vi "checkplayerstatus.vi"(11 "player":T1[](array[typedef]) {"status" items=["host_ready", "idle", "host", "leaved", "ready", "playing", "lose(mine)", "lose(ot)", "win"]}) -> (3 "Numeric":u16, 7 "kick leave":T1[](array[typedef]) {"status" items=["host_ready", "idle", "host", "leaved", "ready", "playing", "lose(mine)", "lose(ot)", "win"]})   [LabVIEW 2025]
uses:
  controls/playerstatus.ctl
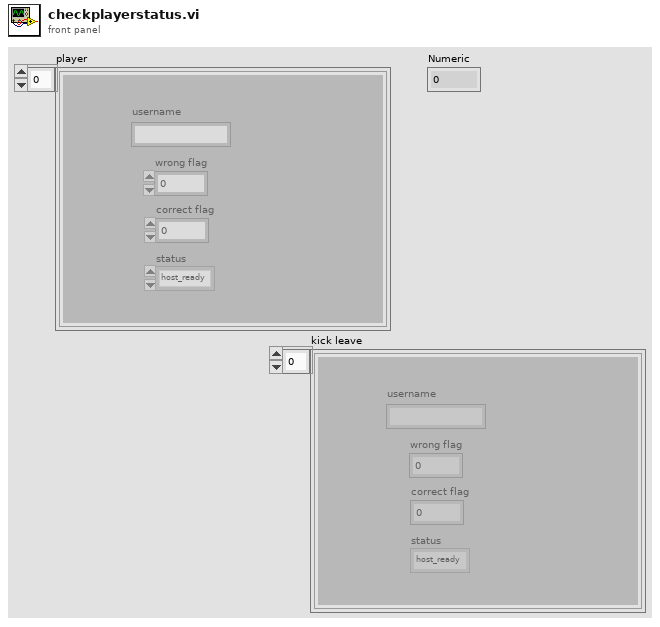
[diagram p1: front panel]
types:
  T1 = typedef "playerstatus.ctl" = cluster{"correct flag":i32, "wrong flag":i32, "username":string, "status":u16}
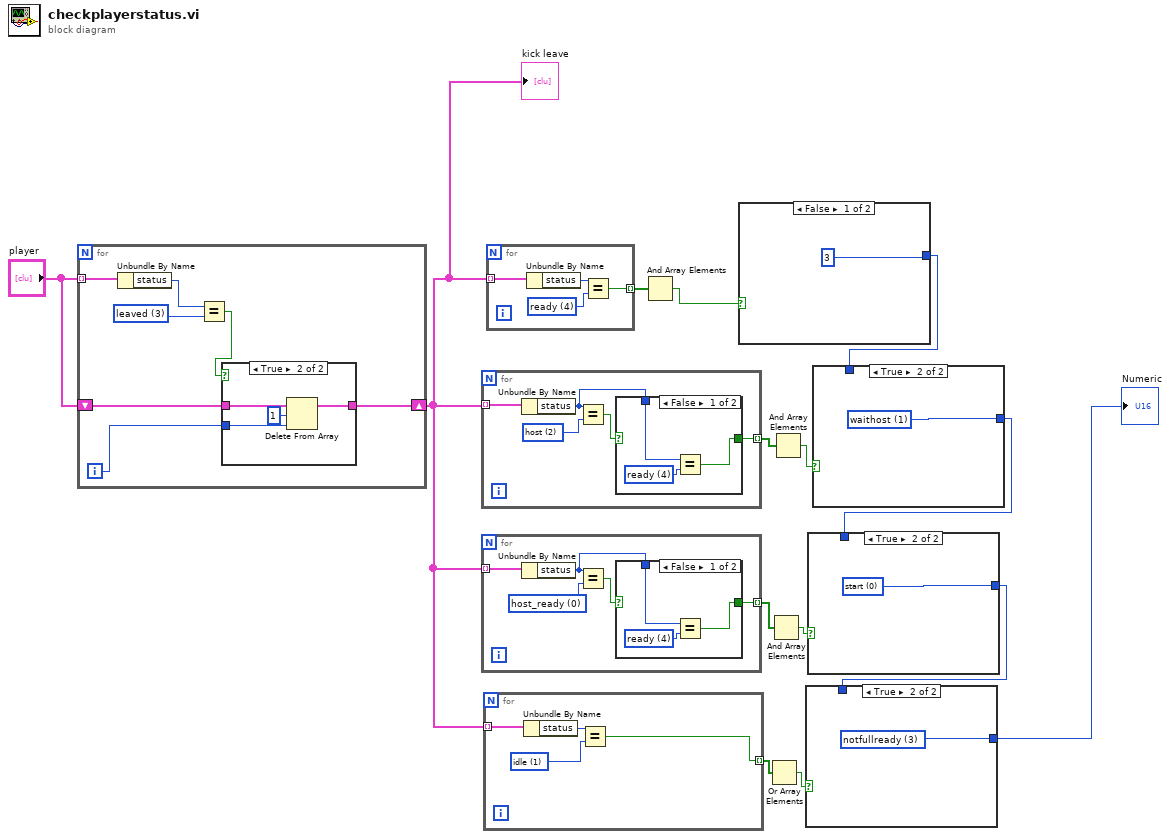
[diagram p0: block diagram]
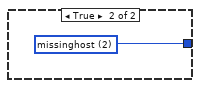
[diagram p7: hidden frame]
diagram:
  n1 = for {
    tunnel: "player" -> [w20] mode=indexing
    shift-right: [w15] -> w1
    shift-left: "player" -> [w18]
    i -> [w16]
    w19 = u16 3 items=["host_ready", "idle", "host", "leaved", "ready", "playing", "lose(mine)", "lose(ot)", "win"] ("status")
    n2 = Unbundle By Name(w20) -> ("status"=w21:u16)
    n3 = Equal?(x=w21, y=w19) -> (x = y?=w17:bool)
    n4 = case shown="True" w17 {
      tunnel: w18 -> [w22 w26]
      tunnel: w16 -> [_ w25]
      tunnel: [w22 w23] -> w15
      frame False {
      }
      frame True {
        n5 = Delete From Array(array=w26, length=1, index=w25) -> (array with subset deleted=w23:T1[])  [unwired: 1 out]
      }
    }
  }
  "kick leave" <- w1
  n6 = for {
    tunnel: w1 -> [w31] mode=indexing
    tunnel: [w28] -> w11 mode=indexing
    w30 = u16 2 items=["host_ready", "idle", "host", "leaved", "ready", "playing", "lose(mine)", "lose(ot)", "win"] ("status")
    n7 = Unbundle By Name(w31) -> ("status"=w27:u16)
    n8 = Equal?(x=w27, y=w30) -> (x = y?=w29:bool)
    n9 = case shown="False" w29 {
      selector: w29 -> [_ w35]
      tunnel: [w32 w35] -> w28
      tunnel: w27 -> [w34 _]
      frame False {
        w33 = u16 4 items=["host_ready", "idle", "host", "leaved", "ready", "playing", "lose(mine)", "lose(ot)", "win"] ("status")
        n10 = Equal?(x=w34, y=w33) -> (x = y?=w32:bool)
      }
      frame True {
      }
    }
  }
  n11 = for {
    tunnel: w1 -> [w40] mode=indexing
    tunnel: [w37] -> w7 mode=indexing
    w39 = u16 0 items=["host_ready", "idle", "host", "leaved", "ready", "playing", "lose(mine)", "lose(ot)", "win"] ("status")
    n12 = Unbundle By Name(w40) -> ("status"=w36:u16)
    n13 = Equal?(x=w36, y=w39) -> (x = y?=w38:bool)
    n14 = case shown="False" w38 {
      selector: w38 -> [_ w44]
      tunnel: [w41 w44] -> w37
      tunnel: w36 -> [w43 _]
      frame False {
        w42 = u16 4 items=["host_ready", "idle", "host", "leaved", "ready", "playing", "lose(mine)", "lose(ot)", "win"] ("status")
        n15 = Equal?(x=w43, y=w42) -> (x = y?=w41:bool)
      }
      frame True {
      }
    }
  }
  n16 = for {
    tunnel: w1 -> [w48] mode=indexing
    tunnel: [w45] -> w5 mode=indexing
    w47 = u16 1 items=["host_ready", "idle", "host", "leaved", "ready", "playing", "lose(mine)", "lose(ot)", "win"] ("status")
    n17 = Unbundle By Name(w48) -> ("status"=w46:u16)
    n18 = Equal?(x=w46, y=w47) -> (x = y?=w45:bool)
  }
  n19 = for {
    tunnel: w1 -> [w52] mode=indexing
    tunnel: [w49] -> w13 mode=indexing
    w50 = u16 4 items=["host_ready", "idle", "host", "leaved", "ready", "playing", "lose(mine)", "lose(ot)", "win"] ("status")
    n20 = Unbundle By Name(w52) -> ("status"=w51:u16)
    n21 = Equal?(x=w51, y=w50) -> (x = y?=w49:bool)
  }
  n22 = And Array Elements(Boolean array=w13) -> (logical AND=w12:bool)
  n23 = case shown="False" w12 {
    tunnel: [u16 3 w54] -> w9
    frame False {
    }
    frame True {
      w54 = u16 2 items=["start", "waithost", "missinghost", "notfullready"]
    }
  }
  n24 = Or Array Elements(Boolean array=w5) -> (logical OR=w4:bool)
  n25 = And Array Elements(Boolean array=w7) -> (logical AND=w6:bool)
  n26 = And Array Elements(Boolean array=w11) -> (logical AND=w10:bool)
  n27 = case shown="True" w10 {
    tunnel: [w55 w56] -> w8
    tunnel: w9 -> [w55 _]
    frame False {
    }
    frame True {
      w56 = u16 1 items=["start", "waithost", "missinghost", "notfullready"]
    }
  }
  n28 = case shown="True" w6 {
    tunnel: [w57 w58] -> w3
    tunnel: w8 -> [w57 _]
    frame False {
    }
    frame True {
      w58 = u16 0 items=["start", "waithost", "missinghost", "notfullready"]
    }
  }
  n29 = case shown="True" w4 {
    tunnel: [w59 w60] -> w2
    tunnel: w3 -> [w59 _]
    frame False {
    }
    frame True {
      w60 = u16 3 items=["start", "waithost", "missinghost", "notfullready"]
    }
  }
  "Numeric" <- w2
